vi "流量计UI.vi"() -> ()   [LabVIEW 2016]
uses:
  <vilib>/Utility/config.llb/NI_LVConfig.lvlib
panel:
  in  "流量计启用":bool[](array[boolean])
  out "累积流量":u32[](array[numeric])
  out "水位":dbl[](array[numeric])
  out "流速":dbl[](array[numeric])
  out "流量":dbl[](array[numeric])
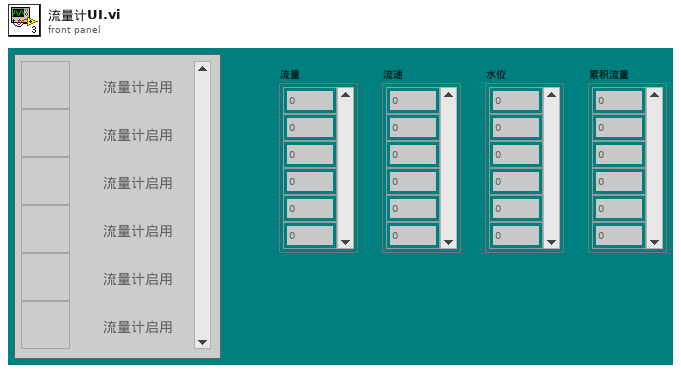
[diagram p1: front panel]
types:
  T1 = typedef "LVDateTimeRec.ctl" = cluster{"秒数的小数部分":dbl, "秒":i32, "分":i32, "时":i32, "日":i32, "月":i32, "年":i32, "天数（周）":i32, "天数（年）":i32, "DST":i32}
  T2 = cluster{"时间标识":timestamp, "监测值":sgl, "单位":string}
  T3 = enum32{"Bad", "Idle", "Run top level", "Running"}
  T4 = typedef "NI_LVConfig.lvlib/Config Data RefNum.ctl" = refnum<k1>
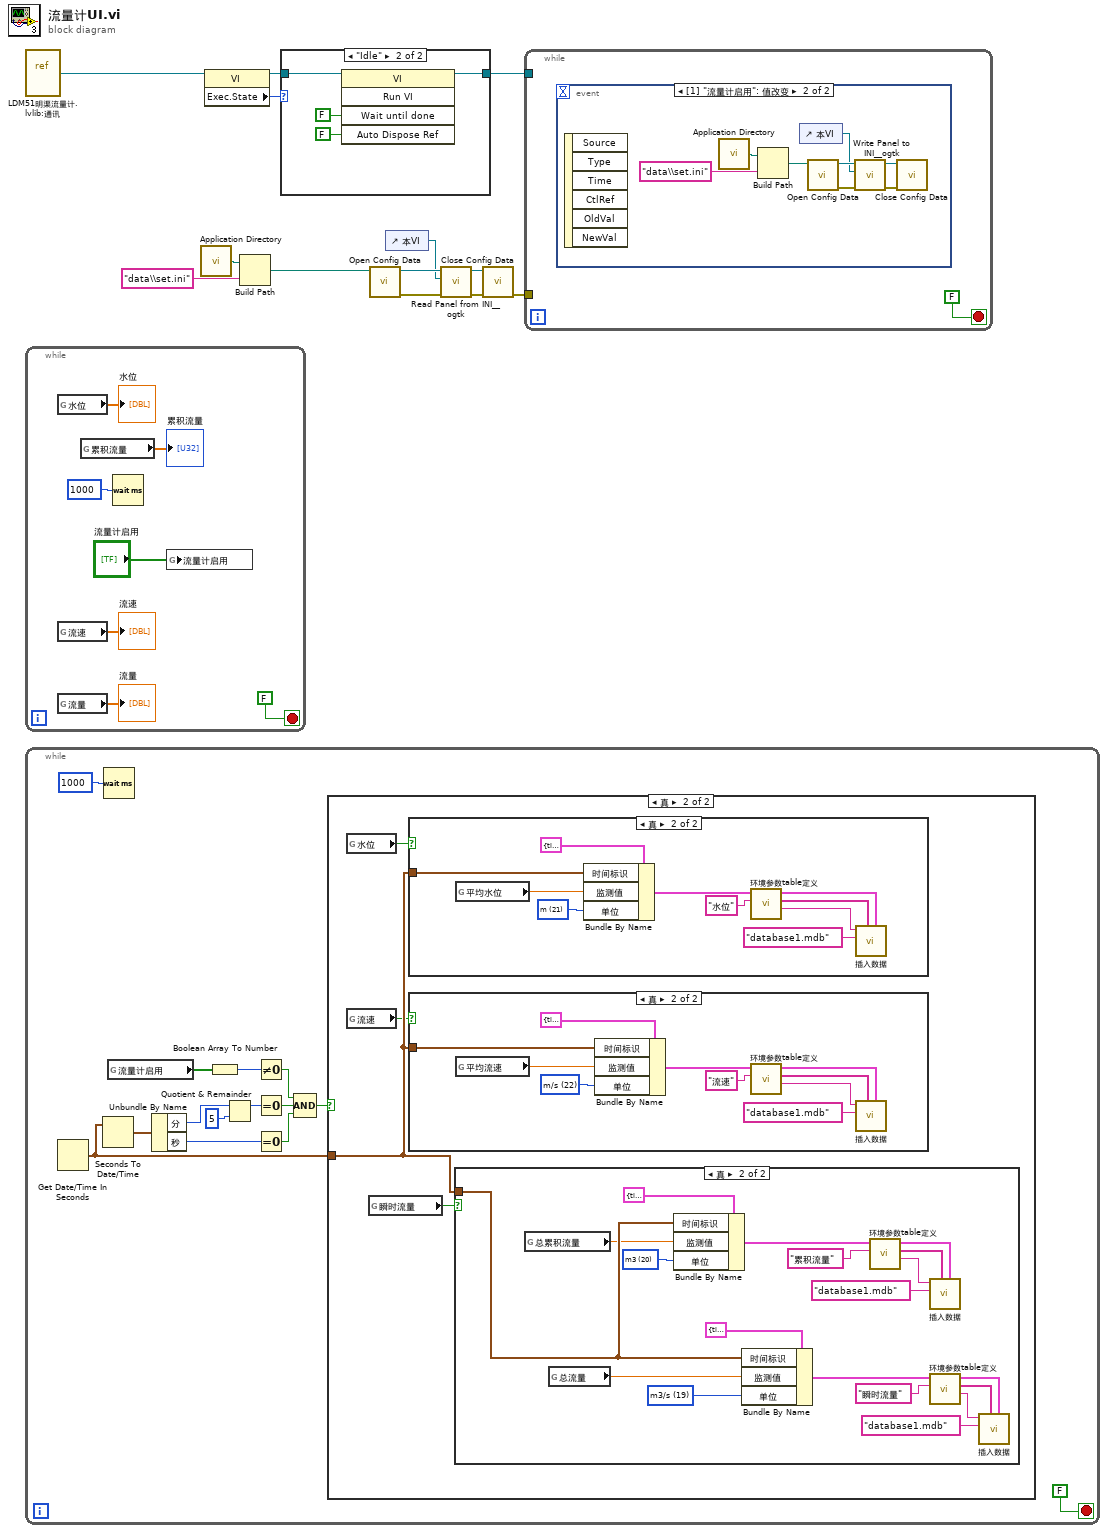
[diagram p0: block diagram]
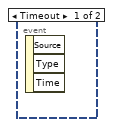
[diagram p7: hidden frame]
diagram:
  n1 = vi-ref "LDM51明渠流量计.lvlib:通讯.vi"() -> (w13:refnum<vi>)
  n2 = while {
    stop <- FALSE stop-if-true
    n3 = global read "LDM51全局变量.vi" "水位"() -> (→"水位":dbl[])
    n4 = global read "LDM51全局变量.vi" "流速"() -> (→"流速":dbl[])
    n5 = global read "LDM51全局变量.vi" "流量"() -> (→"流量":dbl[])
    n6 = global read "LDM51全局变量.vi" "累积流量"() -> (→"累积流量":dbl[])
    n7 = Wait (ms)(milliseconds to wait=u32 1000 ("等待时间（毫秒）")) -> ()  [unwired: 1 out]
    n8 = global write "LDM51全局变量.vi" "流量计启用"("流量计启用") -> ()
  }
  n9 = while {
    stop <- FALSE stop-if-true
    n10 = Get Date/Time In Seconds() -> (seconds since 1Jan1904=w33:timestamp)
    n11 = Seconds To Date/Time(time stamp (now)=w33) -> (date time rec=w32:T1)  [unwired: 1 in]
    n12 = Wait (ms)(milliseconds to wait=u32 1000 ("等待时间（毫秒）")) -> ()  [unwired: 1 out]
    n13 = global read "LDM51全局变量.vi" "流量计启用"() -> (w23:bool[])
    n14 = Unbundle By Name(w32) -> ("分"=w31:i32, "秒"=w29:i32)
    n15 = Boolean Array To Number(Boolean array=w23) -> (number=w22:u32)
    n16 = Quotient & Remainder(x=w31, y=5) -> (x-y*floor(x/y)=w28:i32)  [unwired: 1 out]
    n17 = Not Equal To 0?(x=w22) -> (x != 0?=w21:bool)
    n18 = Equal To 0?(x=w28) -> (x = 0?=w27:bool)
    n19 = Equal To 0?(x=w29) -> (x = 0?=w26:bool)
    n20 = Compound Arithmetic op=AND ("复合运算")(w21, w27, w26) -> (w25:bool)
    n21 = case shown="真" w25 {
      tunnel: w33 -> [_ w38]
      frame False {
      }
      frame True {
        n22 = global read "副屏设置全局变量.vi" "水位"() -> (w37:bool)
        n23 = global read "副屏设置全局变量.vi" "流速"() -> (w36:bool)
        n24 = global read "副屏设置全局变量.vi" "瞬时流量"() -> (w35:bool)
        n25 = case shown="真" w37 {
          tunnel: w38 -> [_ w71]
          frame False {
          }
          frame True {
            w68 = u16 21 items=["ug/L", "mg/L", "ppm", "mg/m3", "cm", "ppb", "ug/m3", "%", "nmol/mol", "umol/mol", "MPN/L", "MPN/100ml", "ng/m3", "NTU", "无量纲", "ms/cm", "us/cm", "℃", "V", "m3/s", "m3", "m", "m/s"] ("单位")
            n26 = global read "LDM51全局变量.vi" "平均水位"() -> (w69:dbl)
            n27 = Bundle By Name(cluster=cluster{"时间标识":timestamp, "监测值":sgl, "单位":u16} {"时间标识"=timestamp(0 s since 1904-01-01), "监测值"=0.0, "单位"=0} ("data"), "时间标识"=w71, "监测值"=w69, "单位"=w68) -> (w74:cluster{"时间标识":timestamp, "监测值":sgl, "单位":u16})
            n28 = call "环境参数table定义.vi"("table 输入"="水位", "data"=w74) -> ("table 输出"=w77:string, "columns"=w76:string[], "data输出"=w75:T2)  [unwired: 7 in]
            n29 = call "插入数据.vi"("data"=w75, "columns"=w76, "database"="database1.mdb" ("table 输入"), "table"=w77) -> ()  [unwired: 7 in, 1 out]
          }
        }
        n30 = case shown="真" w36 {
          tunnel: w38 -> [_ w60]
          frame False {
          }
          frame True {
            w58 = u16 22 items=["ug/L", "mg/L", "ppm", "mg/m3", "cm", "ppb", "ug/m3", "%", "nmol/mol", "umol/mol", "MPN/L", "MPN/100ml", "ng/m3", "NTU", "无量纲", "ms/cm", "us/cm", "℃", "V", "m3/s", "m3", "m", "m/s"] ("单位")
            n31 = global read "LDM51全局变量.vi" "平均流速"() -> (w59:dbl)
            n32 = Bundle By Name(cluster=cluster{"时间标识":timestamp, "监测值":sgl, "单位":u16} {"时间标识"=timestamp(0 s since 1904-01-01), "监测值"=0.0, "单位"=0} ("data"), "时间标识"=w60, "监测值"=w59, "单位"=w58) -> (w65:cluster{"时间标识":timestamp, "监测值":sgl, "单位":u16})
            n33 = call "环境参数table定义.vi"("table 输入"="流速", "data"=w65) -> ("table 输出"=w61:string, "columns"=w62:string[], "data输出"=w63:T2)  [unwired: 7 in]
            n34 = call "插入数据.vi"("data"=w63, "columns"=w62, "database"="database1.mdb" ("table 输入"), "table"=w61) -> ()  [unwired: 7 in, 1 out]
          }
        }
        n35 = case shown="真" w35 {
          tunnel: w38 -> [_ w45]
          frame False {
          }
          frame True {
            w39 = u16 20 items=["ug/L", "mg/L", "ppm", "mg/m3", "cm", "ppb", "ug/m3", "%", "nmol/mol", "umol/mol", "MPN/L", "MPN/100ml", "ng/m3", "NTU", "无量纲", "ms/cm", "us/cm", "℃", "V", "m3/s", "m3", "m", "m/s"] ("单位")
            w41 = u16 19 items=["ug/L", "mg/L", "ppm", "mg/m3", "cm", "ppb", "ug/m3", "%", "nmol/mol", "umol/mol", "MPN/L", "MPN/100ml", "ng/m3", "NTU", "无量纲", "ms/cm", "us/cm", "℃", "V", "m3/s", "m3", "m", "m/s"] ("单位")
            n36 = global read "LDM51全局变量.vi" "总累积流量"() -> (w40:dbl)
            n37 = global read "LDM51全局变量.vi" "总流量"() -> (w42:dbl)
            n38 = Bundle By Name(cluster=cluster{"时间标识":timestamp, "监测值":sgl, "单位":u16} {"时间标识"=timestamp(0 s since 1904-01-01), "监测值"=0.0, "单位"=0} ("data"), "时间标识"=w45, "监测值"=w40, "单位"=w39) -> (w48:cluster{"时间标识":timestamp, "监测值":sgl, "单位":u16})
            n39 = Bundle By Name(cluster=cluster{"时间标识":timestamp, "监测值":sgl, "单位":u16} {"时间标识"=timestamp(0 s since 1904-01-01), "监测值"=0.0, "单位"=0} ("data"), "时间标识"=w45, "监测值"=w42, "单位"=w41) -> (w55:cluster{"时间标识":timestamp, "监测值":sgl, "单位":u16})
            n40 = call "环境参数table定义.vi"("table 输入"="累积流量", "data"=w48) -> ("table 输出"=w51:string, "columns"=w50:string[], "data输出"=w49:T2)  [unwired: 7 in]
            n41 = call "插入数据.vi"("data"=w49, "columns"=w50, "database"="database1.mdb" ("table 输入"), "table"=w51) -> ()  [unwired: 7 in, 1 out]
            n42 = call "环境参数table定义.vi"("table 输入"="瞬时流量", "data"=w55) -> ("table 输出"=w52:string, "columns"=w53:string[], "data输出"=w54:T2)  [unwired: 7 in]
            n43 = call "插入数据.vi"("data"=w54, "columns"=w53, "database"="database1.mdb" ("table 输入"), "table"=w52) -> ()  [unwired: 7 in, 1 out]
          }
        }
      }
    }
  }
  n44 = call <vilib>:"Application Directory.vi"() -> ("Application Directory"=w8:path)
  n45 = property class="VI"(reference=w13) -> (reference out=w12:refnum<vi>, "Exec.State"=w11:T3)  [unwired: 1 in, 1 out]
  n46 = Build Path(base path=w8, name or relative path="data\\set.ini" ("名称或相对路径")) -> (appended path=w9:path)
  n47 = case shown="\"Idle\"" w11 {
    tunnel: w12 -> [w78 w80]
    tunnel: [w78 w79] -> w2
    frame "Bad", Default {
    }
    frame "Idle" {
      n48 = invoke class="VI" method="Run VI"(reference=w80, "Wait until done"=FALSE ("结束前等待"), "Auto Dispose Ref"=FALSE ("自动销毁引用")) -> (reference out=w79:refnum<vi>)  [unwired: 2 in, 4 out]
    }
  }
  n49 = call <vilib>:"Open Config Data.vi"("configuration file path"=w9) -> ("error out"=w6:errorcluster, "refnum"=w7:T4)  [unwired: 8 in, 1 out]
  n50 = control-ref of="本VI"() -> (w5:refnum<vi>)
  n51 = call <userlib>:"Read Panel from INI__ogtk.vi"("error in (no error)"=w6, "VI ref"=w5, "refnum"=w7) -> ("error out"=w3:errorcluster, "refnum out"=w4:T4)  [unwired: 7 in]
  n52 = call <vilib>:"Close Config Data.vi"("error in (no error)"=w3, "refnum"=w4) -> ("error out"=w1:errorcluster)  [unwired: 8 in, 1 out]
  n53 = while {
    tunnel: w2 -> [_]
    tunnel: w1 -> [_]
    stop <- FALSE stop-if-true
    n54 = event shown="[1] \"流量计启用\": 值改变" {
      selector: _ -> [_ _]
      dyn-events: _ -> [_ _]
      timeout: _ -> [_ _]
      event Timeout {
        n55 = event-data() -> ()  [unwired: 1 in, 3 out]
      }
      event "流量计启用": Value Change {
        n56 = event-data() -> ()  [unwired: 1 in, 6 out]
        n57 = call <vilib>:"Application Directory.vi"() -> ("Application Directory"=w86:path)
        n58 = Build Path(base path=w86, name or relative path="data\\set.ini" ("名称或相对路径")) -> (appended path=w85:path)
        n59 = control-ref of="本VI"() -> (w87:refnum<vi>)
        n60 = call <vilib>:"Open Config Data.vi"("configuration file path"=w85) -> ("error out"=w89:errorcluster, "refnum"=w91:T4)  [unwired: 8 in, 1 out]
        n61 = call <userlib>:"Write Panel to INI__ogtk.vi"("error in (no error)"=w89, "VI ref"=w87, "refnum"=w91) -> ("error out"=w88:errorcluster, "refnum out"=w90:T4)  [unwired: 7 in]
        n62 = call <vilib>:"Close Config Data.vi"("error in (no error)"=w88, "refnum"=w90) -> ()  [unwired: 8 in, 2 out]
      }
    }
  }
